vi "mainScanner.vi"(8 "Error In":errorcluster, 11 "scanUDE":T1) -> (0 "Error Out":errorcluster)   [LabVIEW 2018]
uses:
  controls/scanUDE.ctl
  Controller Module/src/controls/controllerData.ctl
  UI Module/src/controls/mainAppElementsCluster.ctl
  Modbus Module/src/controls/modbusData.ctl
  controls/readRegisterModbusCluster.ctl
  Barcode Printer Module/src/controls/printData.ctl
  controls/scanData.ctl
  controls/serialPortEnum.ctl
panel:
  out "Read Value":string
  in  "Scan":bool
  in  "OK":bool
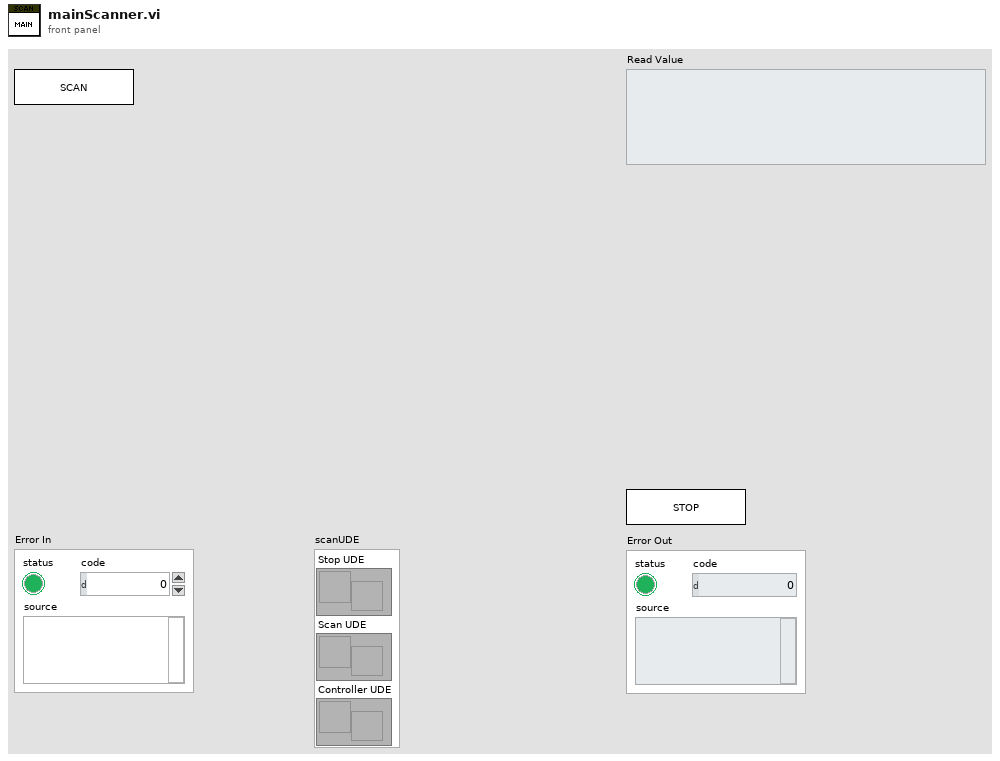
[diagram p1: front panel]
types:
  T1 = typedef "scanUDE.ctl" = cluster{"Stop UDE":refnum<user-event>, "Controller UDE":refnum<user-event>, "Scan UDE":refnum<user-event>}
  T2 = enum32{"Invalid", "Standard", "Closed", "Hidden", "Minimized", "Maximized"}
  T3 = enum32{"invalid app kind", "Development System", "Run Time System", "Student Edition", "Embedded LabVIEW", "Evaluation", "Custom"}
  T4 = typedef "serialPortEnum.ctl" = enum16{"init", "write", "read", "close"}
  T5 = cluster{"Core":cluster{"Current VI Reference":refnum<vi>, "Close Panel on Exit?":bool}, "Com Port":refnum<visa-resource-name>, "Scanned QR":string}
  T6 = cluster{"Current VI Reference":refnum<vi>, "Close Panel on Exit?":bool}
  T7 = typedef "pathCluster.ctl" = cluster{"src Folder Path":path, "Controller Module Path":path, "UI Module Path":path, "Model Select Module Path":path, "Barcode Printer Module Path":path, "Barcode Scanner Module Path":path, "Database Module Path":path, "Report Generation Path":path, "Simulation Path":path, "subVIs Folder Path":path, "info Folder Path":path, "config file Path":path, "cutomerLogo Path":path, "database File Path":path}
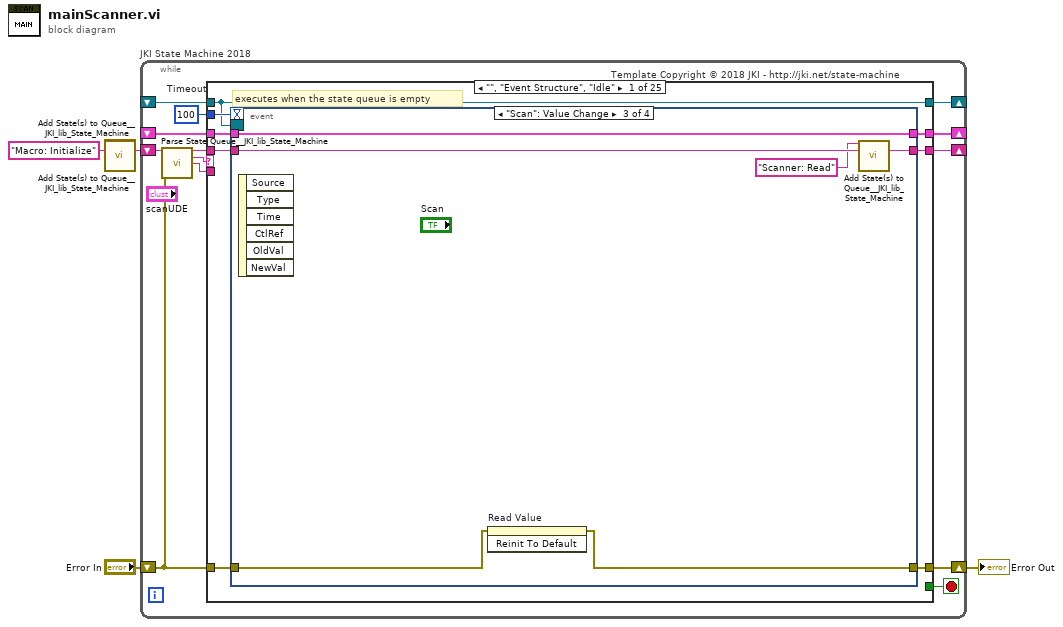
[diagram p0: block diagram]
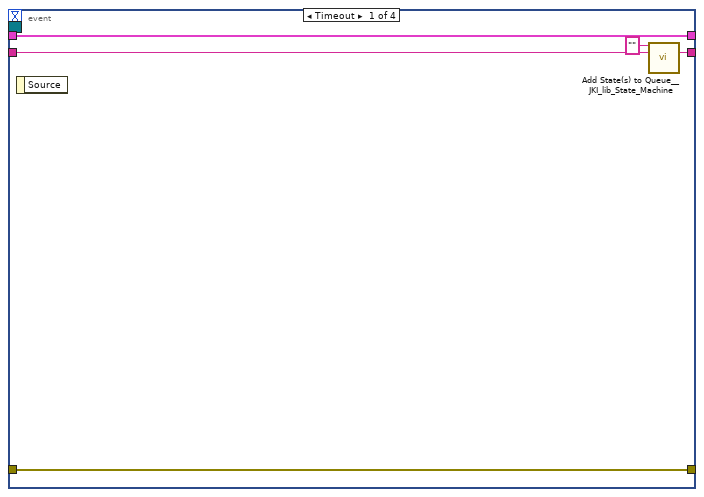
[diagram p2: hidden frame]
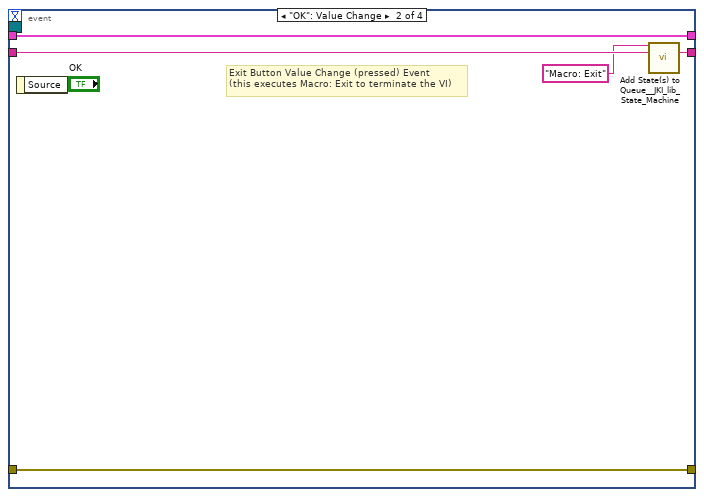
[diagram p3: hidden frame]
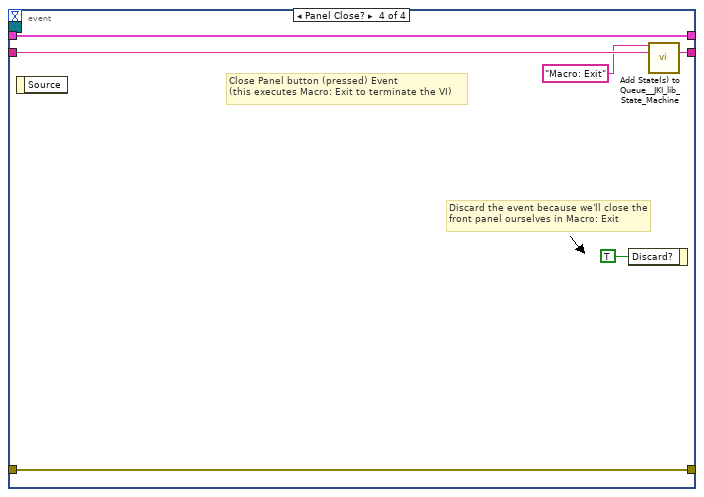
[diagram p4: hidden frame]
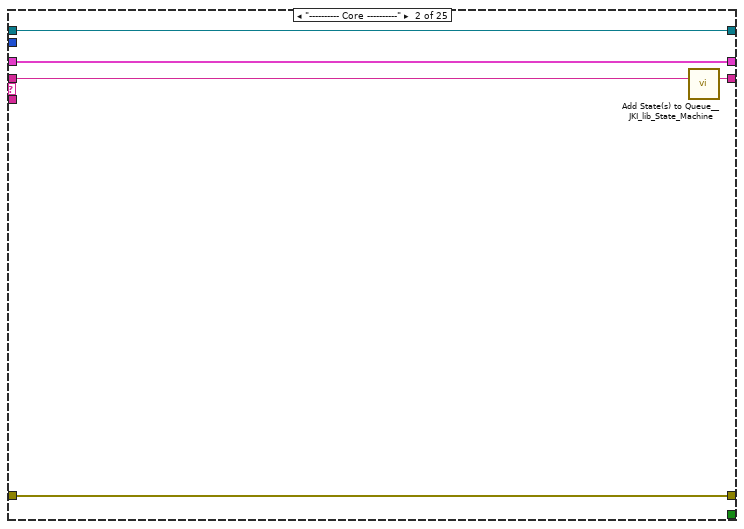
[diagram p5: hidden frame]
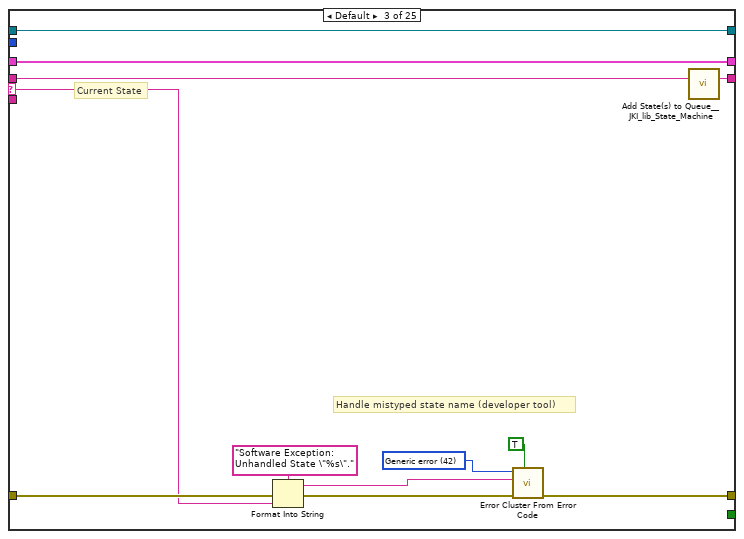
[diagram p6: hidden frame]
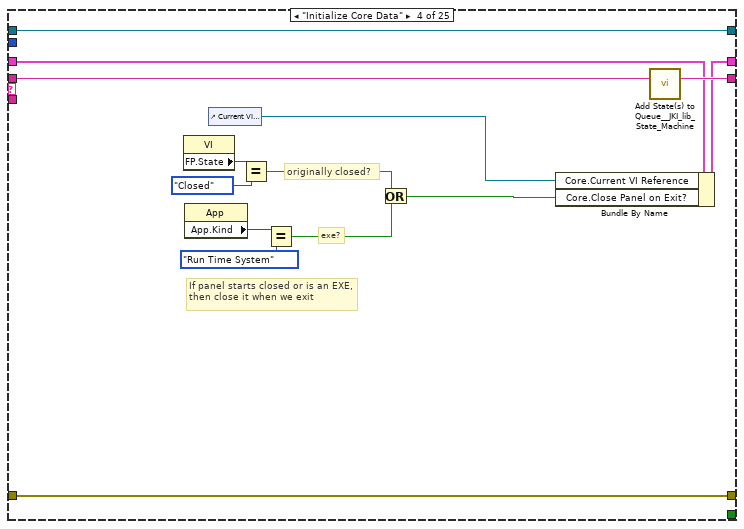
[diagram p7: hidden frame]
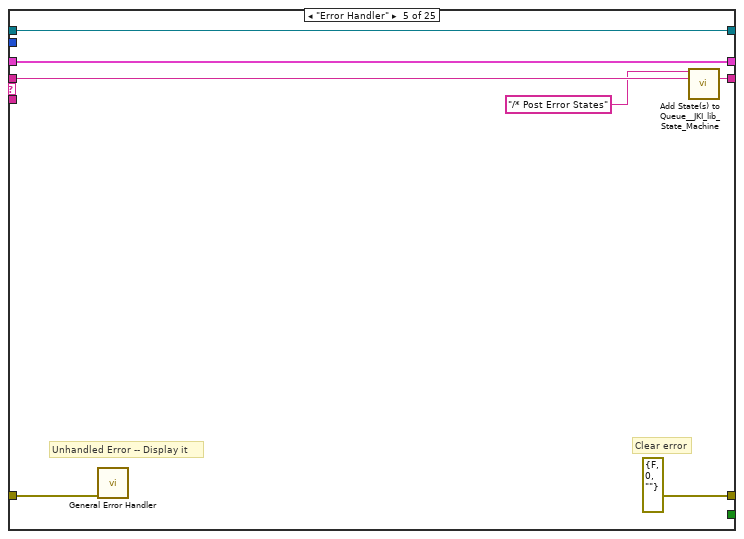
[diagram p8: hidden frame]
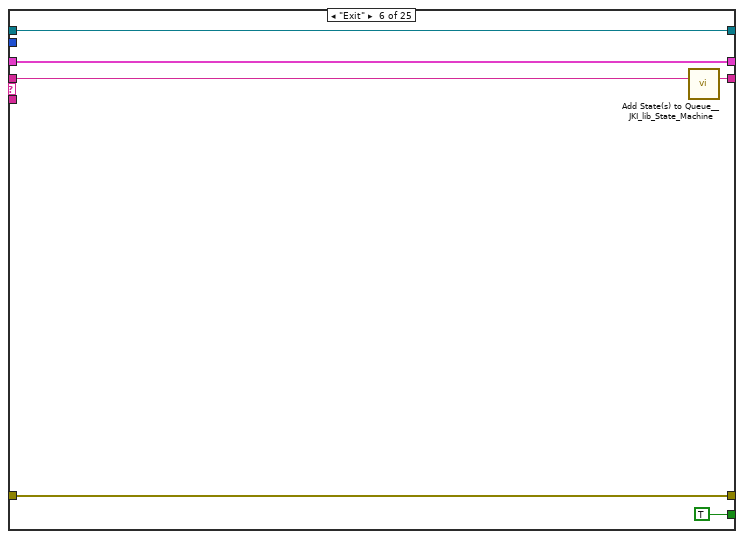
[diagram p9: hidden frame]
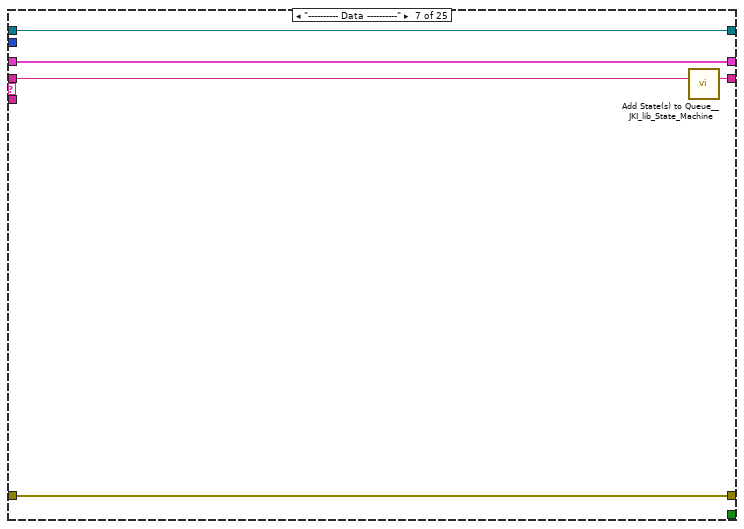
[diagram p10: hidden frame]
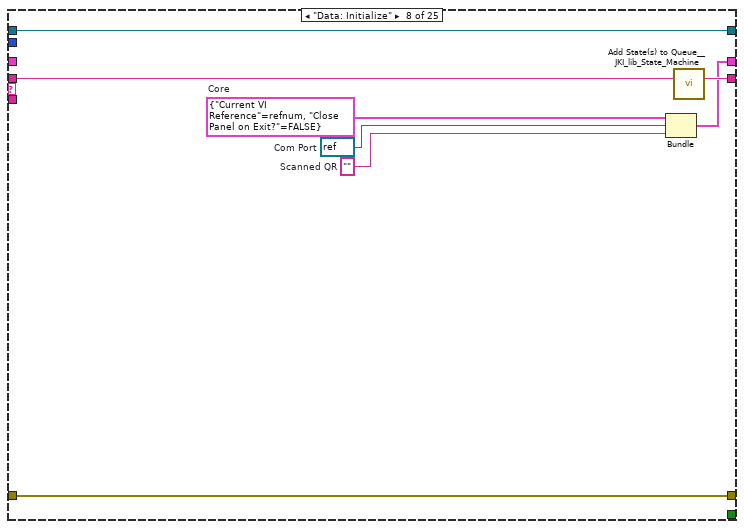
[diagram p11: hidden frame]
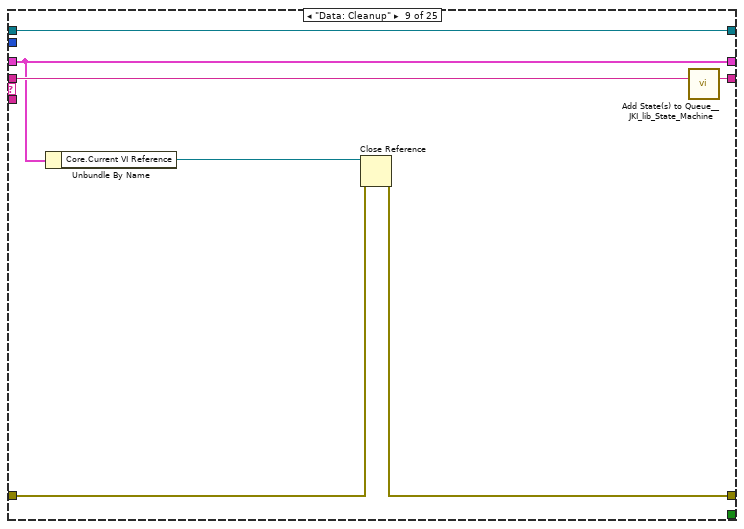
[diagram p12: hidden frame]
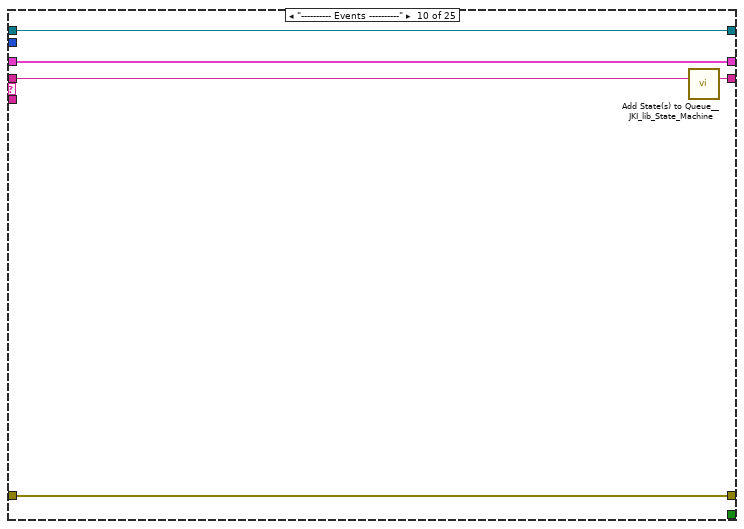
[diagram p13: hidden frame]
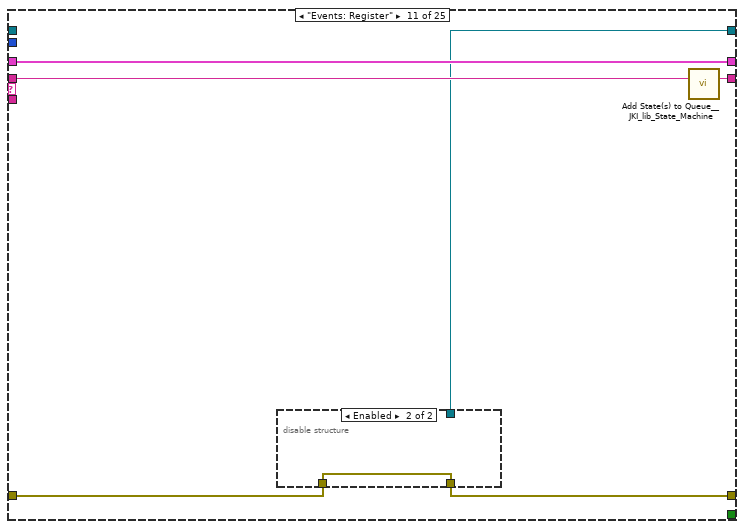
[diagram p14: hidden frame]
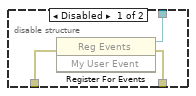
[diagram p15: hidden frame]
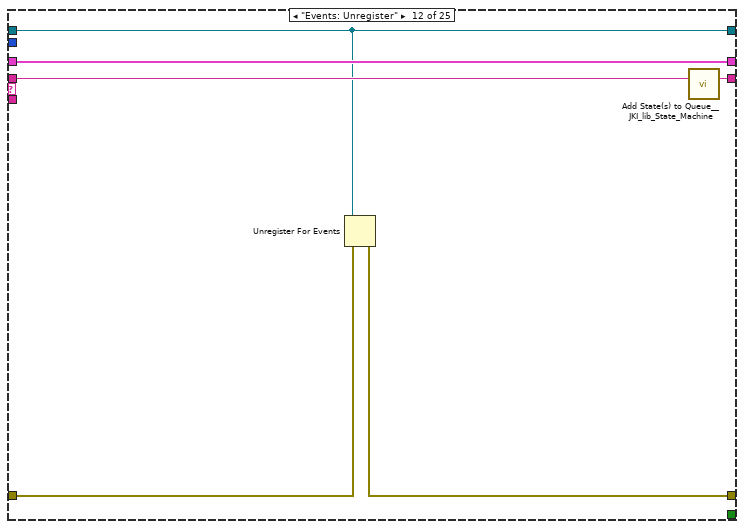
[diagram p16: hidden frame]
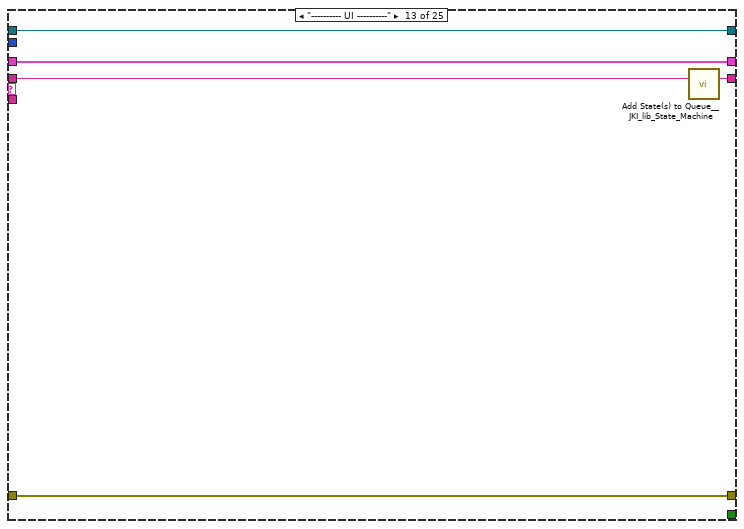
[diagram p17: hidden frame]
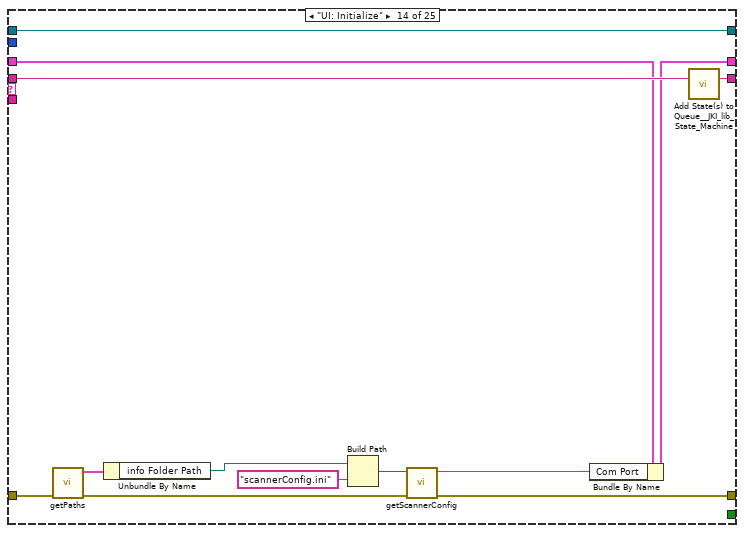
[diagram p18: hidden frame]
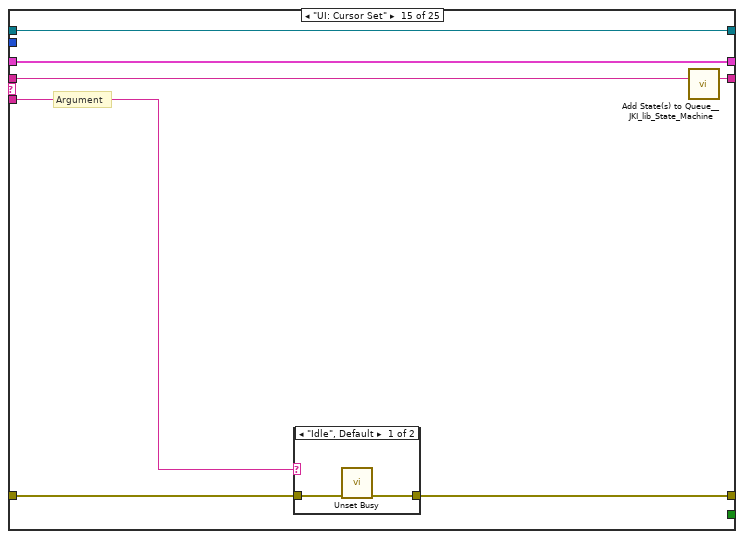
[diagram p19: hidden frame]
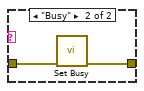
[diagram p20: hidden frame]
diagram:
  n1 = call <vilib>:"Add State(s) to Queue__JKI_lib_State_Machine.vi"() -> ()  [unwired: 15 in, 1 out]
  n2 = call <vilib>:"Add State(s) to Queue__JKI_lib_State_Machine.vi"("State(s) in (\"\")"="Macro: Initialize") -> ("States Out"=w4:string)  [unwired: 14 in]
  n3 = while "JKI State Machine 2018" {
    shift-right: [w10] -> _
    shift-left: _ -> [w9]
    shift-right: [w13] -> w2
    shift-left: "Error In" -> [w7]
    shift-right: [w12] -> _
    shift-left: w4 -> [w14]
    shift-right: [w6] -> _
    shift-left: _ -> [w5]
    stop <- w11 stop-if-true
    w8 = 100  # Timeout
    # "Template Copyright © 2018 JKI - http://jki.net/state-machine"
    n4 = call <vilib>:"Parse State Queue__JKI_lib_State_Machine.vi"("State Queue"=w14, "Error In (no error)"=w7) -> ("Remaining States"=w16:string, "Current State"=w17:string, "Arguments"=w15:string)  [unwired: 11 in]
    n5 = case shown="\"\", \"Event Structure\", \"Idle\"" w17 {
      selector: w17 -> [_ _ w54 _ _ _ _ _ _ _ _ _ _ _ _ _ _ _ _ _ _ _ _ _ _]
      tunnel: w16 -> [w25 w52 w58 w78 w85 w91 w96 w104 w111 w116 w122 w132 w137 w150 w157 w169 w239 w245 w256 w261 w269 w284 w291 w296 w302]
      tunnel: w15 -> [_ _ _ _ _ _ _ _ _ _ _ _ _ _ w152 w163 _ _ _ _ _ _ _ _ _]
      tunnel: w9 -> [w23 w49 w56 w71 w82 w89 w93 _ w106 w113 w120 w130 w134 w140 w155 w165 w236 w242 w253 w258 w263 w276 w289 w293 w298]
      tunnel: [w22 w50 w60 w75 errorcluster {"status"=FALSE, "code"=0, "source"=""} ("error out") w88 w94 w101 w107 w114 w118 w127 w135 w142 w153 w166 w237 w243 w254 w259 w265 w278 w286 w294 w300] -> w13
      tunnel: w7 -> [w21 w50 w59 w75 w81 w88 w94 w101 w108 w114 w117 w128 w135 w147 w154 w167 w237 w243 w254 w259 w266 w281 w287 w294 w300]
      tunnel: [w24 w51 w57 w77 w84 w90 w95 w103 w110 w115 w121 w131 w136 w149 w156 w168 w238 w244 w255 w260 w268 w283 w290 w295 w301] -> w12
      tunnel: [_ _ _ _ _ TRUE _ _ _ _ _ _ _ _ _ _ _ _ _ _ _ _ _ _ _] -> w11
      tunnel: [w20 w49 w56 w76 w82 w89 w93 w102 w106 w113 w120 w130 w134 w139 w155 w165 w236 w242 w253 w258 w263 w275 w289 w293 w298] -> w10
      tunnel: w8 -> [w19 _ _ _ _ _ _ _ _ _ _ _ _ _ _ _ _ _ _ _ _ _ _ _ _]
      tunnel: [w18 w48 w53 w65 w79 w86 w92 w99 w105 w112 w119 w129 w133 w148 w151 w162 w235 w240 w246 w257 w267 w282 w288 w292 w299] -> w6
      tunnel: w5 -> [w18 w48 w53 w65 w79 w86 w92 w99 w105 w112 _ w129 w133 w148 w151 w162 w235 w240 w246 w257 w267 w282 w288 w292 w299]
      frame "", "Event Structure", "Idle" {
        # "executes when the state queue is empty"
        n6 = event shown="[2] \"Scan\": Value Change" {
          selector: w18 -> [_ _ _ _]
          dyn-events: _ -> [_ _ _ _]
          timeout: w19 -> [_ _ _ _]
          tunnel: w25 -> [w30 w35 w40 w47]
          tunnel: [w29 w34 w39 w46] -> w24
          tunnel: w23 -> [w27 w32 w41 w44]
          tunnel: [w28 w33 w36 w45] -> w22
          tunnel: w21 -> [w28 w33 w37 w45]
          tunnel: [w27 w32 w41 w44] -> w20
          event Timeout {
            n7 = event-data() -> ()  [unwired: 1 in, 1 out]
            n8 = call <vilib>:"Add State(s) to Queue__JKI_lib_State_Machine.vi"("State(s) in Front (\"\")"="" ("State(s) in Front (\"\")"), "State(s) in (\"\")"=w30) -> ("States Out"=w29:string)  [unwired: 13 in]
          }
          event "OK": Value Change {
            # "Exit Button Value Change (pressed) Event\n(this executes Macro: Exit to terminate the VI)"
            n9 = event-data() -> ()  [unwired: 1 in, 1 out]
            n10 = call <vilib>:"Add State(s) to Queue__JKI_lib_State_Machine.vi"("State(s) in Front (\"\")"="Macro: Exit", "State(s) in (\"\")"=w35) -> ("States Out"=w34:string)  [unwired: 13 in]
          }
          event "Scan": Value Change {
            n11 = event-data() -> ()  [unwired: 1 in, 6 out]
            n12 = invoke on="Read Value" class="Str" method="Reinit To Default"(error in=w37) -> (error out=w36:errorcluster)  [unwired: 2 in, 2 out]
            n13 = call <vilib>:"Add State(s) to Queue__JKI_lib_State_Machine.vi"("State(s) in Front (\"\")"="Scanner: Read" ("State(s) in Front (\"\")"), "State(s) in (\"\")"=w40) -> ("States Out"=w39:string)  [unwired: 13 in]
          }
          event Panel Close? {
            # "Discard the event because we'll close the front panel ourselves in Macro: Exit"
            # "Close Panel button (pressed) Event\n(this executes Macro: Exit to terminate the VI)"
            n14 = event-data() -> ()  [unwired: 1 in, 1 out]
            n15 = event-data("Discard?"=TRUE) -> ()  [unwired: 1 in, 1 out]
            n16 = call <vilib>:"Add State(s) to Queue__JKI_lib_State_Machine.vi"("State(s) in Front (\"\")"="Macro: Exit", "State(s) in (\"\")"=w47) -> ("States Out"=w46:string)  [unwired: 13 in]
          }
        }
      }
      frame "---------- Core ----------" {
        n17 = call <vilib>:"Add State(s) to Queue__JKI_lib_State_Machine.vi"("State(s) in (\"\")"=w52) -> ("States Out"=w51:string)  [unwired: 14 in]
      }
      frame Default {
        w63 = 42 items=["No error", "Argument error", "Memory is full", "Out of zone", "End of file", "File already open", "Generic file I/O error", "File not found", "File permission error", "Disk is full", "Duplicate path", "Too many files open", "System feature not enabled", "Resource file not found", "Cannot add resource", "Resource not found", "Image not found", "Image memory error", "Pen does not exist", "Config type invalid", "Config token not found", "Config parse error", "Config memory error", "Bad external code format", "Bad external code offset", "External code not present", "Null window", "Destroy window error", "Null menu", "Print aborted", "Bad print record", "Print driver error", "Windows error during printing", "Memory error during printing", "Print dialog error", "Generic print error", "Invalid device refnum", "Device not found", "Device parameter error", "Device unit error", "Cannot open device", "Device call aborted", "Generic error", "Cancelled by user", "Object ID too low", "Object ID too high", "Object not in heap", "Unknown heap", "Unknown object (invalid DefProc)", "Unknown object (DefProc not in table)", "Message out of range", "Invalid (null) method", "Unknown message", "Manager call not supported", "Bad address", "Network operation in progress", "Network operation timed out", "Connection is busy", "Network attribute not supported", "Network error", "Address in use", "System out of memory", "Connection aborted", "Connection refused", "Not connected", "Already connected", "Connection closed", "Initialization error (interapplication manager)", "Bad occurrence", "Wait on unbound occurrence handler", "Occurrence queue overflow", "Datalog type conflict", "Unused", "Unrecognized type (interapplication manager)", "Memory corrupt", "Failed to make temporary DLL", "Old CIN version", "Drag socket not found", "Failed to load drop-object", "Failed to register OLE object", "Failed to release OLE object", "Format specifier type mismatch", "Unknown format specifier", "Too few format specifiers", "Too many format specifiers", "Scan failed", "Newer CIN version", "Error converting to variant", "Runtime menu error", "Password tampered", "Variant attribute not found", "Incompatible variant data type", "Event data is not available", "Event Store is not present", "Occurrence is not found", "Event Queue is not created", "Event info is not available", "Refnum passed is NULL", "Error retrieving Class GUID", "Error retrieving CoClass GUID", "Error retrieving TypeLib GUID.", "Bad built application magic bytes.", "Specific driver is different from the specific driver associated with the Logical Name.", "There is no session opened to the class driver.", "Max Error", "MAX - Error with config objects", "MAX - Error loading configuration", "MAX - Group not supported"]
        # "Current State"
        # "Handle mistyped state name (developer tool)"
        n18 = Format Into String(format string="Software Exception: Unhandled State \"%s\"." ("message"), error in=w59, w54) -> (resulting string=w62:string, error out=w61:errorcluster)  [unwired: 1 in]
        n19 = call <vilib>:"Error Cluster From Error Code.vi"("show call chain? (False)"=TRUE, "error in (no error)"=w61, "error message (\"\")"=w62, "error code (0)"=w63) -> ("error out"=w60:errorcluster)  [unwired: 5 in]
        n20 = call <vilib>:"Add State(s) to Queue__JKI_lib_State_Machine.vi"("State(s) in (\"\")"=w58) -> ("States Out"=w57:string)  [unwired: 14 in]
      }
      frame "Initialize Core Data" {
        # "originally closed?"
        # "exe?"
        # "If panel starts closed or is an EXE, then close it when we exit"
        n21 = property class="VI"() -> ("FP.State"=w68:T2)  [unwired: 2 in, 2 out]
        n22 = property class="App"() -> ("App.Kind"=w74:T3)  [unwired: 2 in, 2 out]
        n23 = control-ref of="Current VI Reference"() -> (w69:refnum<vi>)
        n24 = Equal?(x=w68, y=T2."Closed" ("Front Panel Window:State")) -> (x = y?=w66:bool)
        n25 = Equal?(x=w74, y=T3."Run Time System" ("Application:Kind")) -> (x = y?=w72:bool)
        n26 = Or(x=w66, y=w72) -> (x .or. y?=w70:bool)
        n27 = Bundle By Name(cluster=w71, "Core.Current VI Reference"=w69, "Core.Close Panel on Exit?"=w70) -> (w76:T5)
        n28 = call <vilib>:"Add State(s) to Queue__JKI_lib_State_Machine.vi"("State(s) in (\"\")"=w78) -> ("States Out"=w77:string)  [unwired: 14 in]
      }
      frame "Error Handler" {
        # "Unhandled Error -- Display it"
        # "Clear error"
        n29 = call <vilib>:"General Error Handler.vi"("error in (no error)"=w81) -> ()  [unwired: 10 in, 5 out]
        n30 = call <vilib>:"Add State(s) to Queue__JKI_lib_State_Machine.vi"("State(s) in Front (\"\")"="/* Post Error States", "State(s) in (\"\")"=w85) -> ("States Out"=w84:string)  [unwired: 13 in]
      }
      frame "Exit" {
        n31 = call <vilib>:"Add State(s) to Queue__JKI_lib_State_Machine.vi"("State(s) in (\"\")"=w91) -> ("States Out"=w90:string)  [unwired: 14 in]
      }
      frame "---------- Data ----------" {
        n32 = call <vilib>:"Add State(s) to Queue__JKI_lib_State_Machine.vi"("State(s) in (\"\")"=w96) -> ("States Out"=w95:string)  [unwired: 14 in]
      }
      frame "Data: Initialize" {
        w97 = ""  # Scanned QR
        w98 = refnum<visa-resource-name> refnum  # Com Port
        w100 = T6 {"Current VI Reference"=refnum, "Close Panel on Exit?"=FALSE}  # Core
        n33 = Bundle("Core"=w100, "Com Port"=w98, "Scanned QR"=w97) -> (w102:T5)  [unwired: 1 in]
        n34 = call <vilib>:"Add State(s) to Queue__JKI_lib_State_Machine.vi"("State(s) in (\"\")"=w104) -> ("States Out"=w103:string)  [unwired: 14 in]
      }
      frame "Data: Cleanup" {
        n35 = Unbundle By Name(w106) -> ("Core.Current VI Reference"=w109:refnum<vi>)
        n36 = Close Reference(reference=w109, error in (no error)=w108) -> (error out=w107:errorcluster)
        n37 = call <vilib>:"Add State(s) to Queue__JKI_lib_State_Machine.vi"("State(s) in (\"\")"=w111) -> ("States Out"=w110:string)  [unwired: 14 in]
      }
      frame "---------- Events ----------" {
        n38 = call <vilib>:"Add State(s) to Queue__JKI_lib_State_Machine.vi"("State(s) in (\"\")"=w116) -> ("States Out"=w115:string)  [unwired: 14 in]
      }
      frame "Events: Register" {
        n39 = disable-structure shown="Enabled" {
          disable-tunnel: [w125 _] -> w119
          disable-tunnel: [w124 w126] -> w118
          disable-tunnel: w117 -> [w123 w126]
          frame Disabled {
            n40 = register-events(error in=w123) -> (reference out=w125:refnum<event-registration>, error out=w124:errorcluster)  [unwired: 2 in]
          }
          frame Enabled {
          }
        }
        n41 = call <vilib>:"Add State(s) to Queue__JKI_lib_State_Machine.vi"("State(s) in (\"\")"=w122) -> ("States Out"=w121:string)  [unwired: 14 in]
      }
      frame "Events: Unregister" {
        n42 = Unregister For Events(event registration refnum=w129, error in=w128) -> (error out=w127:errorcluster)
        n43 = call <vilib>:"Add State(s) to Queue__JKI_lib_State_Machine.vi"("State(s) in (\"\")"=w132) -> ("States Out"=w131:string)  [unwired: 14 in]
      }
      frame "---------- UI ----------" {
        n44 = call <vilib>:"Add State(s) to Queue__JKI_lib_State_Machine.vi"("State(s) in (\"\")"=w137) -> ("States Out"=w136:string)  [unwired: 14 in]
      }
      frame "UI: Initialize" {
        n45 = call "getPaths.vi"("Error In"=w147) -> ("Error Out"=w143:errorcluster, "Application Path Cluster"=w146:T7)  [unwired: 9 in]
        n46 = Unbundle By Name(w146) -> ("info Folder Path"=w145:path)
        n47 = Build Path(base path=w145, name or relative path="scannerConfig.ini") -> (appended path=w141:path)
        n48 = call "getScannerConfig.vi"("Error In"=w143, "Config File Path"=w141) -> ("Error Out"=w142:errorcluster, "comPort"=w138:string)  [unwired: 8 in]
        n49 = Bundle By Name(cluster=w140, "Com Port"=w138) -> (w139:T5)
        n50 = call <vilib>:"Add State(s) to Queue__JKI_lib_State_Machine.vi"("State(s) in (\"\")"=w150) -> ("States Out"=w149:string)  [unwired: 14 in]
      }
      frame "UI: Cursor Set" {
        # "Argument"
        n51 = case shown="\"Idle\", Default" w152 {
          tunnel: w154 -> [w159 w161]
          tunnel: [w158 w160] -> w153
          frame "Idle", Default {
            n52 = call <vilib>:"Unset Busy.vi"("error in (no error)"=w159) -> ("error out"=w158:errorcluster)  [unwired: 10 in]
          }
          frame "Busy" {
            n53 = call <vilib>:"Set Busy.vi"("error in (no error)"=w161) -> ("error out"=w160:errorcluster)  [unwired: 9 in, 1 out]
          }
        }
        n54 = call <vilib>:"Add State(s) to Queue__JKI_lib_State_Machine.vi"("State(s) in (\"\")"=w157) -> ("States Out"=w156:string)  [unwired: 14 in]
      }
      frame "UI: Front Panel State" {
        # "Argument"
        n55 = Unbundle By Name(w165) -> ("Core.Current VI Reference"=w164:refnum<vi>)
        n56 = case shown="\"Minimize\", \"Minimized\"" w163 {
          tunnel: w167 -> [w175 w190 w201 w214 w227]
          tunnel: [w177 w191 w203 w216 w229] -> w166
          tunnel: w164 -> [w176 w188 w202 w215 w228]
          frame "Open", "Standard", Default {
            w170 = T2."Standard" ("State")
            n57 = property class="VI"(reference=w176, error in=w175) -> (reference out=w173:refnum<vi>, error out=w174:errorcluster, "FP.State"=w172:T2)
            n58 = Not Equal?(x=w172, y=w170) -> (x != y?=w171:bool)
            n59 = case shown="True" w171 {
              tunnel: [w181 w183] -> w177
              tunnel: w174 -> [w180 w183]
              tunnel: w173 -> [w179 _]
              tunnel: w170 -> [w178 _]
              frame True {
                n60 = invoke class="VI" method="FP.Open"(reference=w179, error in=w180, "Activate"=TRUE, "State"=w178) -> (error out=w181:errorcluster)  [unwired: 1 in, 4 out]
              }
              frame False {
              }
            }
          }
          frame "Close", "Closed" {
            n61 = property class="VI"(reference=w188, error in=w190) -> (reference out=w187:refnum<vi>, error out=w189:errorcluster, "FP.State"=w185:T2)
            n62 = Not Equal?(x=w185, y=T2."Closed" ("Front Panel Window:State")) -> (x != y?=w184:bool)
            n63 = case shown="True" w184 {
              tunnel: [w192 w195] -> w191
              tunnel: w189 -> [w192 w194]
              tunnel: w187 -> [_ w193]
              frame False {
              }
              frame True {
                n64 = invoke class="VI" method="FP.Close"(reference=w193, error in=w194) -> (error out=w195:errorcluster)  [unwired: 1 in, 2 out]
              }
            }
          }
          frame "Hidden", "Hide" {
            w196 = T2."Hidden" ("State")
            n65 = property class="VI"(reference=w202, error in=w201) -> (reference out=w199:refnum<vi>, error out=w200:errorcluster, "FP.State"=w198:T2)
            n66 = Not Equal?(x=w198, y=w196) -> (x != y?=w197:bool)
            n67 = case shown="True" w197 {
              tunnel: [w207 w208] -> w203
              tunnel: w200 -> [w206 w208]
              tunnel: w199 -> [w205 _]
              tunnel: w196 -> [w204 _]
              frame True {
                n68 = invoke class="VI" method="FP.Open"(reference=w205, error in=w206, "State"=w204) -> (error out=w207:errorcluster)  [unwired: 2 in, 4 out]
              }
              frame False {
              }
            }
          }
          frame "Minimize", "Minimized" {
            w209 = T2."Minimized" ("State")
            n69 = property class="VI"(reference=w215, error in=w214) -> (reference out=w212:refnum<vi>, error out=w213:errorcluster, "FP.State"=w211:T2)
            n70 = Not Equal?(x=w211, y=w209) -> (x != y?=w210:bool)
            n71 = case shown="True" w210 {
              tunnel: [w220 w221] -> w216
              tunnel: w213 -> [w219 w221]
              tunnel: w212 -> [w218 _]
              tunnel: w209 -> [w217 _]
              frame True {
                n72 = invoke class="VI" method="FP.Open"(reference=w218, error in=w219, "State"=w217) -> (error out=w220:errorcluster)  [unwired: 2 in, 4 out]
              }
              frame False {
              }
            }
          }
          frame "Maximize", "Maximized" {
            w222 = T2."Maximized" ("State")
            n73 = property class="VI"(reference=w228, error in=w227) -> (reference out=w225:refnum<vi>, error out=w226:errorcluster, "FP.State"=w224:T2)
            n74 = Not Equal?(x=w224, y=w222) -> (x != y?=w223:bool)
            n75 = case shown="True" w223 {
              tunnel: [w233 w234] -> w229
              tunnel: w226 -> [w232 w234]
              tunnel: w225 -> [w231 _]
              tunnel: w222 -> [w230 _]
              frame True {
                n76 = invoke class="VI" method="FP.Open"(reference=w231, error in=w232, "State"=w230) -> (error out=w233:errorcluster)  [unwired: 2 in, 4 out]
              }
              frame False {
              }
            }
          }
        }
        n77 = call <vilib>:"Add State(s) to Queue__JKI_lib_State_Machine.vi"("State(s) in (\"\")"=w169) -> ("States Out"=w168:string)  [unwired: 14 in]
      }
      frame "---------- Macro ----------" {
        n78 = call <vilib>:"Add State(s) to Queue__JKI_lib_State_Machine.vi"("State(s) in (\"\")"=w239) -> ("States Out"=w238:string)  [unwired: 14 in]
      }
      frame "Macro: Initialize" {
        n79 = call <vilib>:"Add State(s) to Queue__JKI_lib_State_Machine.vi"("State(s) in Front (\"\")"="Data: Initialize\nInitialize Core Data\nEvents: Register\nUI: Initialize\nScanner: Initialize\nUI: Front Panel State >> Open", "State(s) in (\"\")"=w245) -> ("States Out"=w244:string)  [unwired: 13 in]
      }
      frame "Macro: Exit" {
        n80 = Unbundle By Name(w253) -> ("Core.Close Panel on Exit?"=w252:bool)
        n81 = Select(t="UI: Front Panel State >> Close", s=w252, f="") -> (s? t:f=w249:string)
        n82 = call <vilib>:"Add State(s) to Queue__JKI_lib_State_Machine.vi"("State(s) in (\"\")"=w249, "State(s) at Back (\"\")"="Scanner: Close\nData: Cleanup\nEvents: Unregister\nExit") -> ("States Out"=w247:string)  [unwired: 13 in]
        n83 = call <vilib>:"Add State(s) to Queue__JKI_lib_State_Machine.vi"("State(s) in Front (\"\")"=w247, "State(s) in (\"\")"=w256) -> ("States Out"=w255:string)  [unwired: 13 in]
      }
      frame "---------- Scanner ----------" {
        n84 = call <vilib>:"Add State(s) to Queue__JKI_lib_State_Machine.vi"("State(s) in (\"\")"=w261) -> ("States Out"=w260:string)  [unwired: 14 in]
      }
      frame "Scanner: Initialize" {
        n85 = Unbundle By Name(w263) -> ("Com Port"=w262:refnum<visa-resource-name>)
        n86 = call "serialDriver.vi"("Serial Port Enum"=serialPortEnum."init", "Error In"=w266, "VISA resource name"=w262) -> ("Error Out"=w265:errorcluster)  [unwired: 7 in, 1 out]
        n87 = call <vilib>:"Add State(s) to Queue__JKI_lib_State_Machine.vi"("State(s) in (\"\")"=w269) -> ("States Out"=w268:string)  [unwired: 14 in]
      }
      frame "Scanner: Read" {
        n88 = call "serialDriver.vi"("Serial Port Enum"=serialPortEnum."read", "Error In"=w281) -> ("Error Out"=w279:errorcluster, "Value Out"=w277:string)  [unwired: 8 in]
        n89 = call "verifyQR.vi"("Error In"=w279, "Value In"=w277) -> ("Error Out"=w278:errorcluster, "isValid?"=w273:bool, "Value Out"=w274:string)  [unwired: 7 in]
        n90 = Bundle By Name(cluster=w276, "Scanned QR"=w274) -> (w275:T5)
        n91 = Select(t="Display: Scanned QR" ("State(s) in Front (\"\")"), s=w273, f="Scanner: Read" ("State(s) in Front (\"\")")) -> (s? t:f=w270:string)
        n92 = call <vilib>:"Add State(s) to Queue__JKI_lib_State_Machine.vi"("State(s) in Front (\"\")"=w270, "State(s) in (\"\")"=w284) -> ("States Out"=w283:string)  [unwired: 13 in]
      }
      frame "Scanner: Close" {
        n93 = call "serialDriver.vi"("Serial Port Enum"=serialPortEnum."close", "Error In"=w287) -> ("Error Out"=w286:errorcluster)  [unwired: 8 in, 1 out]
        n94 = call <vilib>:"Add State(s) to Queue__JKI_lib_State_Machine.vi"("State(s) in (\"\")"=w291) -> ("States Out"=w290:string)  [unwired: 14 in]
      }
      frame "---------- Display ----------" {
        n95 = call <vilib>:"Add State(s) to Queue__JKI_lib_State_Machine.vi"("State(s) in (\"\")"=w296) -> ("States Out"=w295:string)  [unwired: 14 in]
      }
      frame "Display: Scanned QR" {
        n96 = Unbundle By Name(w298) -> ("Scanned QR"=→"Read Value":string)
        n97 = call <vilib>:"Add State(s) to Queue__JKI_lib_State_Machine.vi"("State(s) in (\"\")"=w302) -> ("States Out"=w301:string)  [unwired: 14 in]
      }
    }
  }
  "Error Out" <- w2
